vi "DriveConfigConvert.vi"(4 "Static Drive Configuration in":T1={"Correction Gain % (CG)"=1, "Dead Band (DB)"=10, "Dead Band Window (DW)"=10, "Encoder Resolution (ER)"=4000, "Step Mode  (FSB)"=1, "Position Maintenance (FSC)"=0, "Stop on Stall (FSD)"=1, "Activate OP1 on stall (FSE)"=0, "Stop on Trigger 3 (FSF)"=0, "OP2 in Deadband (FSG)"=0, "Stall Detect (FSH)"=1, "Limit Disable (LD)"=0, "Motor Resolution (MR)"=enum."20000", "Limit Switch Sense (OSA)"=0, "Home Position (OSB)"=1, "Home Switch Sense (OSC)"=0, "Encoder Z for Home (OSD)"=1, "Reference edge of Home (OSH)"=0, "RS232 Echo Control (SSA)"=0, "Buffer at Limit (SSG)"=1, "Buffer at Stop (SSH)"=1, "Indexer Mode  (FSA)"=1, "Type"="", "ConfigString"="", "De Power Motor"=enum."FALSE"} {"Indexer Mode  (FSA)" items=["Incremental", "Absolute"]; "Buffer at Stop (SSH)" items=["Clear buffer", "Save and Continue"]; "Buffer at Limit (SSG)" items=["Clear buffer", "Save and Continue"]; "RS232 Echo Control (SSA)" items=["Echo ON", "Echo OFF"]; "Reference edge of Home (OSH)" items=["CW", "CCW"]; "Encoder Z for Home (OSD)" items=["Don't use", "Enable"]; "Home Switch Sense (OSC)" items=["Normally Open", "Normally Closed"]; "Home Position (OSB)" items=["Anywhere in Switch", "Edge of Switch"]; "Limit Switch Sense (OSA)" items=["Normally Closed", "Normally Open"]; "Limit Disable (LD)" items=["Both Enabled", "CW Disabled", "CCW Disabled", "Both Disabled"]; "Stall Detect (FSH)" items=["Disable", "Enable"]; "OP2 in Deadband (FSG)" items=["Don't Use", "ACTIVATE"]; "Stop on Trigger 3 (FSF)" items=["Ignore", "STOP!"]; "Activate OP1 on stall (FSE)" items=["Do not Activate", "ACTIVATE!"]; "Stop on Stall (FSD)" items=["Continue", "STOP"]; "Position Maintenance (FSC)" items=["Disabled", "Enabled"]; "Step Mode  (FSB)" items=["Motor", "Encoder"]; "Encoder Resolution (ER)" min=1 max=50000; "Dead Band Window (DW)" min=0 max=999999999; "Dead Band (DB)" min=0 max=999999999; "Correction Gain % (CG)" items=["n/a", "12.5", "25", "37.5", "50", "62.5", "75", "87.5", "100"]}, 5 "Values in":string[](array[string]), 6 "Ch names In":string[](array[string]), 7 "Mode":enum16{"Cluster to String", "String to Cluster"}(ring)) -> (0 "Static Drive Configuration Out":T1={"Correction Gain % (CG)"=1, "Dead Band (DB)"=10, "Dead Band Window (DW)"=10, "Encoder Resolution (ER)"=4000, "Step Mode  (FSB)"=1, "Position Maintenance (FSC)"=0, "Stop on Stall (FSD)"=1, "Activate OP1 on stall (FSE)"=0, "Stop on Trigger 3 (FSF)"=0, "OP2 in Deadband (FSG)"=0, "Stall Detect (FSH)"=1, "Limit Disable (LD)"=0, "Motor Resolution (MR)"=enum."20000", "Limit Switch Sense (OSA)"=0, "Home Position (OSB)"=1, "Home Switch Sense (OSC)"=0, "Encoder Z for Home (OSD)"=1, "Reference edge of Home (OSH)"=0, "RS232 Echo Control (SSA)"=0, "Buffer at Limit (SSG)"=1, "Buffer at Stop (SSH)"=1, "Indexer Mode  (FSA)"=1, "Type"="", "ConfigString"="", "De Power Motor"=enum."FALSE"} {"Indexer Mode  (FSA)" items=["Incremental", "Absolute"]; "Buffer at Stop (SSH)" items=["Clear buffer", "Save and Continue"]; "Buffer at Limit (SSG)" items=["Clear buffer", "Save and Continue"]; "RS232 Echo Control (SSA)" items=["Echo ON", "Echo OFF"]; "Reference edge of Home (OSH)" items=["CW", "CCW"]; "Encoder Z for Home (OSD)" items=["Don't use", "Enable"]; "Home Switch Sense (OSC)" items=["Normally Open", "Normally Closed"]; "Home Position (OSB)" items=["Anywhere in Switch", "Edge of Switch"]; "Limit Switch Sense (OSA)" items=["Normally Closed", "Normally Open"]; "Limit Disable (LD)" items=["Both Enabled", "CW Disabled", "CCW Disabled", "Both Disabled"]; "Stall Detect (FSH)" items=["Disable", "Enable"]; "OP2 in Deadband (FSG)" items=["Don't Use", "ACTIVATE"]; "Stop on Trigger 3 (FSF)" items=["Ignore", "STOP!"]; "Activate OP1 on stall (FSE)" items=["Do not Activate", "ACTIVATE!"]; "Stop on Stall (FSD)" items=["Continue", "STOP"]; "Position Maintenance (FSC)" items=["Disabled", "Enabled"]; "Step Mode  (FSB)" items=["Motor", "Encoder"]; "Encoder Resolution (ER)" min=1 max=50000; "Dead Band Window (DW)" min=0 max=999999999; "Dead Band (DB)" min=0 max=999999999; "Correction Gain % (CG)" items=["n/a", "12.5", "25", "37.5", "50", "62.5", "75", "87.5", "100"]}, 1 "String Values":string[](array[string]), 2 "Ch names":string[](array[string]), 3 "Pulses/Rev":i32)   [LabVIEW 2010]
uses:
  DriveStaticConfig.ctl
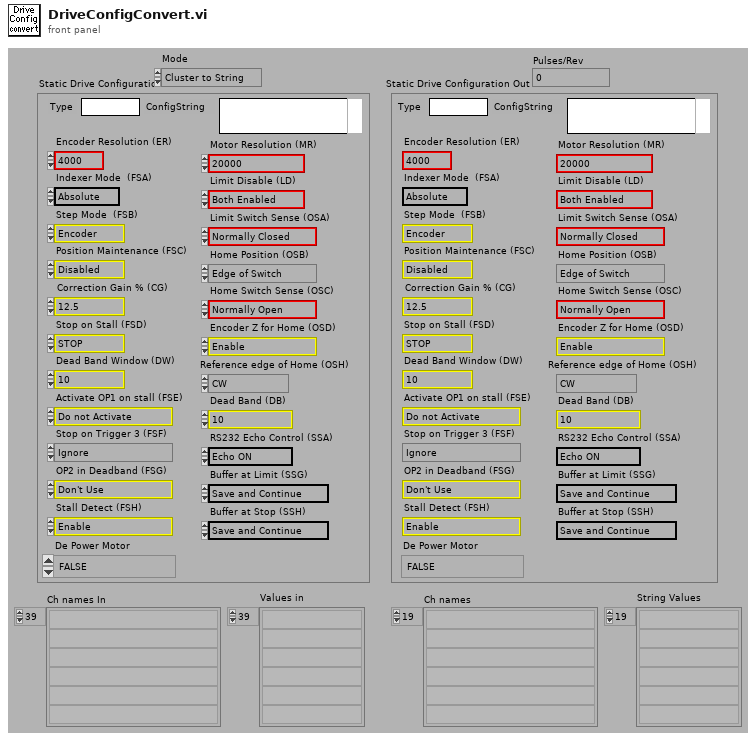
[diagram p1: front panel]
types:
  T1 = typedef "DriveStaticConfig.ctl" = cluster{"Correction Gain % (CG)":u16, "Dead Band (DB)":i32, "Dead Band Window (DW)":i32, "Encoder Resolution (ER)":i32, "Step Mode  (FSB)":u16, "Position Maintenance (FSC)":u16, "Stop on Stall (FSD)":u16, "Activate OP1 on stall (FSE)":u16, "Stop on Trigger 3 (FSF)":u16, "OP2 in Deadband (FSG)":u16, "Stall Detect (FSH)":u16, "Limit Disable (LD)":u16, "Motor Resolution (MR)":enum16{"200", "400", "1000", "2000", "4000", "5000", "10000", "12800", "18000", "20000", "21600", "25000", "25400", "25600", "36000", "50000", "278528", "425984", "507904", "614400", "655360", "819200", "1024000"}, "Limit Switch Sense (OSA)":u16, "Home Position (OSB)":u16, "Home Switch Sense (OSC)":u16, "Encoder Z for Home (OSD)":u16, "Reference edge of Home (OSH)":u16, "RS232 Echo Control (SSA)":u16, "Buffer at Limit (SSG)":u16, "Buffer at Stop (SSH)":u16, "Indexer Mode  (FSA)":u16, "Type":string, "ConfigString":string, "De Power Motor":enum16{"TRUE", "FALSE"}}
  T2 = enum16{"200", "400", "1000", "2000", "4000", "5000", "10000", "12800", "18000", "20000", "21600", "25000", "25400", "25600", "36000", "50000", "278528", "425984", "507904", "614400", "655360", "819200", "1024000"}
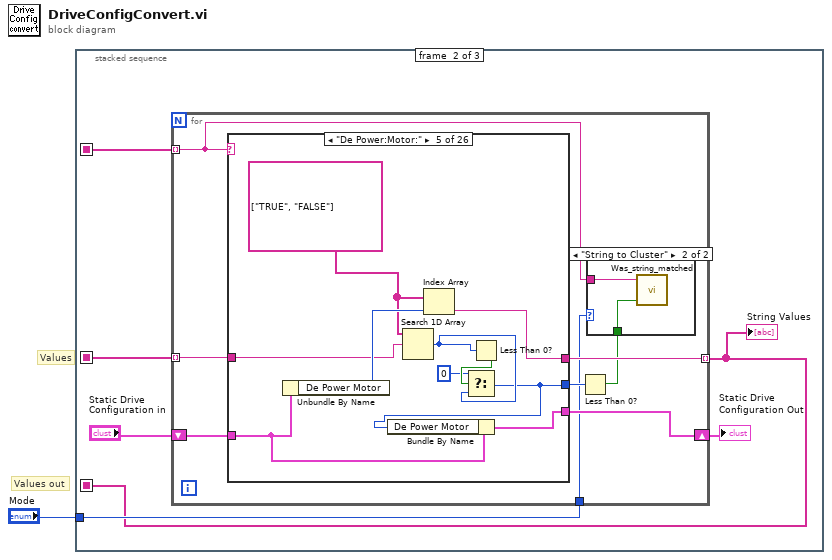
[diagram p0: block diagram]
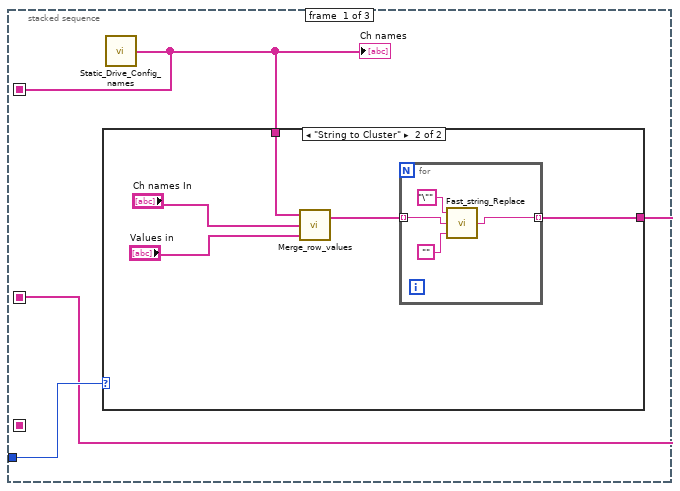
[diagram p2: hidden frame]
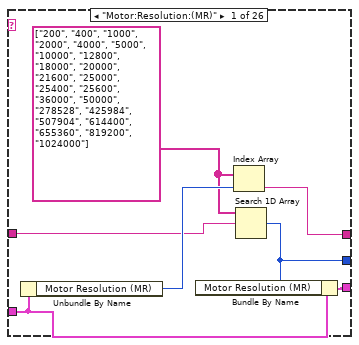
[diagram p5: hidden frame]
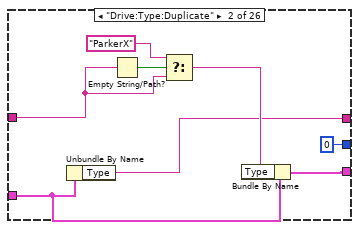
[diagram p6: hidden frame]
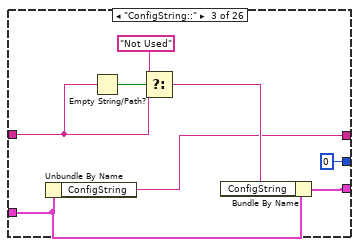
[diagram p7: hidden frame]
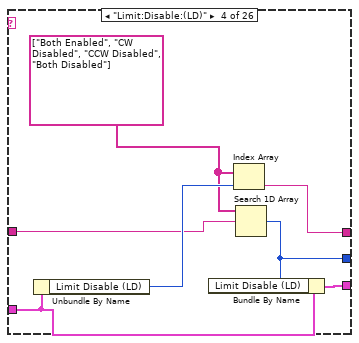
[diagram p8: hidden frame]
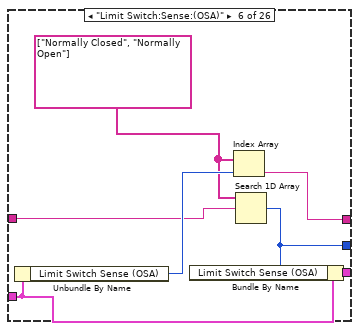
[diagram p9: hidden frame]
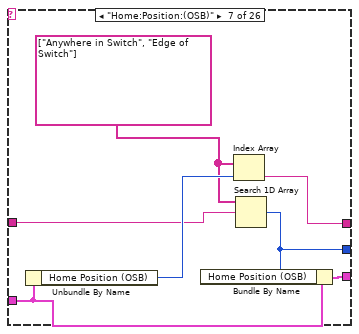
[diagram p10: hidden frame]
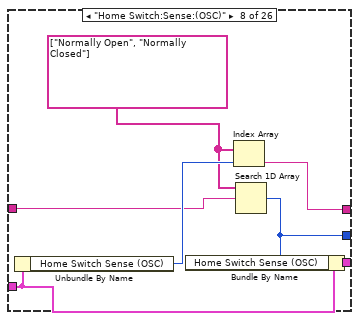
[diagram p11: hidden frame]
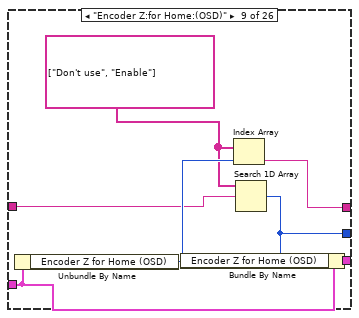
[diagram p12: hidden frame]
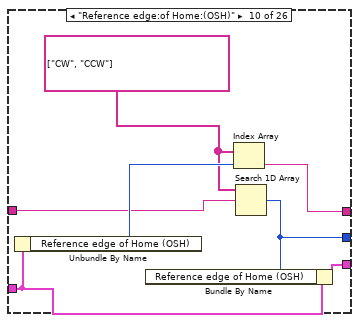
[diagram p13: hidden frame]
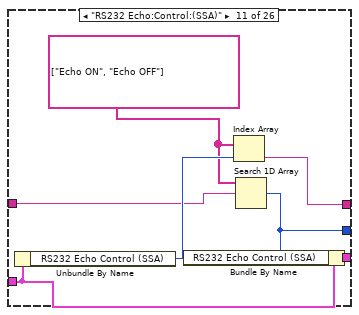
[diagram p14: hidden frame]
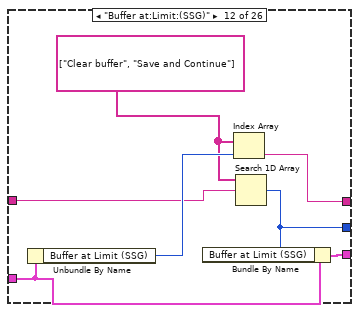
[diagram p15: hidden frame]
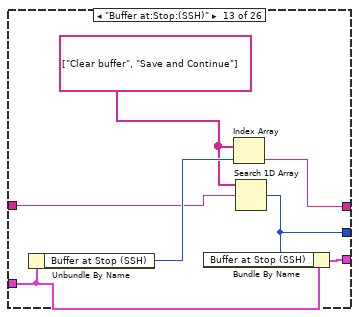
[diagram p16: hidden frame]
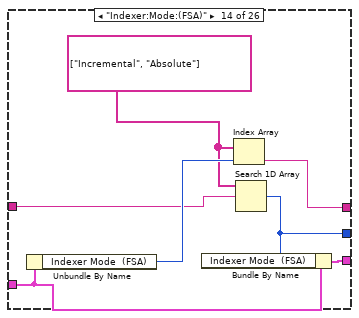
[diagram p17: hidden frame]
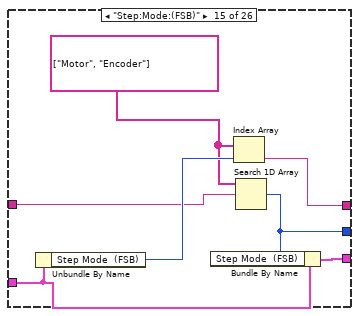
[diagram p18: hidden frame]
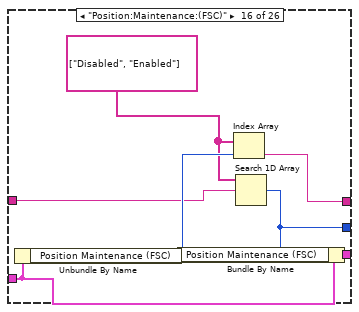
[diagram p19: hidden frame]
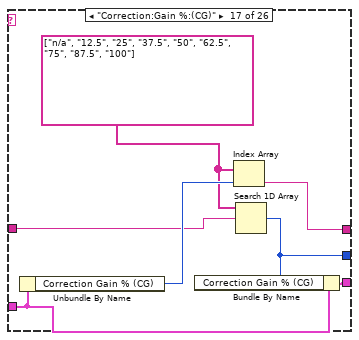
[diagram p20: hidden frame]
diagram:
  # "Values out"
  # "Values"
  n1 = stacked-sequence {
    seq-local: [w3 _ _] -> [_ w17 w222]
    seq-local: [w2 _ _] -> [_ w16 w216]
    seq-local: [_ w15 _] -> [_ _ w223]
    tunnel: "Mode" -> [w4 w18 w225]
    frame #0 {
      n2 = call "Static_Drive_Config_names.vi"() -> ("Ch names"=w2:string[])
      "Ch names" <- w2
      n3 = case shown="\"String to Cluster\"" w4 {
        tunnel: [w5 w6] -> w3
        tunnel: w2 -> [w5 w8]
        frame "Cluster to String" {
        }
        frame "String to Cluster" {
          n4 = call "Merge_row_values.vi"("Present Row values"="Values in", "Present Channels"="Ch names In", "Desired Channels"=w8) -> ("Desired Row values"=w7:string[])  [unwired: 1 out]
          n5 = for {
            tunnel: w7 -> [w14] mode=indexing
            tunnel: [w13] -> w6 mode=indexing
            n6 = call "Fast_string_Replace.vi"("Replace match with:"="", "Input String"=w14, "regular expression"="\"") -> ("Output String"=w13:string)  [unwired: 2 out]
          }
        }
      }
    }
    frame #1 {
      n7 = for {
        tunnel: w16 -> [w22] mode=indexing
        shift-right: [w25] -> w19
        shift-left: "Static Drive Configuration in" -> [w28]
        tunnel: [w27] -> w15 mode=indexing
        tunnel: w17 -> [w26] mode=indexing
        tunnel: w18 -> [w21]
        n8 = case shown="\"De Power:Motor:\"" w22 {
          tunnel: w28 -> [w37 w45 w53 w60 w70 w77 w84 w91 w98 w105 w112 w119 w126 w133 w140 w147 w154 w161 w168 w175 w182 w189 w194 w201 w208 w212]
          tunnel: [w35 w38 w47 w58 w68 w75 w82 w89 w96 w103 w110 w117 w124 w131 w138 w145 w152 w159 w166 w173 w180 w187 w195 w202 w209 ""] -> w27
          tunnel: w26 -> [w34 w41 w50 w57 w67 w74 w81 w88 w95 w102 w109 w116 w123 w130 w137 w144 w151 w158 w165 w172 w179 w186 w192 w199 w206 _]
          tunnel: [w33 w44 w52 w56 w66 w73 w80 w87 w94 w101 w108 w115 w122 w129 w136 w143 w150 w157 w164 w171 w178 w185 w193 w200 w207 w212] -> w25
          tunnel: [w32 0 ("index of element") 0 ("index of element") w55 w61 w72 w79 w86 w93 w100 w107 w114 w121 w128 w135 w142 w149 w156 w163 w170 w177 w184 0 ("index of element") 0 ("index of element") 0 ("index of element") -1 ("index of element")] -> w24
          frame "Motor:Resolution:(MR)" {
            w31 = string[] ["200", "400", "1000", "2000", "4000", "5000", "10000", "12800", "18000", "20000", "21600", "25000", "25400", "25600", "36000", "50000", "278528", "425984", "507904", "614400", "655360", "819200", "1024000"] ("Write Attribute")
            n9 = Unbundle By Name(w37) -> ("Motor Resolution (MR)"=w36:T2)
            n10 = Index Array(array=w31, index=w36) -> (element=w35:string)
            n11 = Search 1D Array(1D array=w31, element=w34) -> (index of element=w32:i32)  [unwired: 1 out]
            n12 = Bundle By Name(cluster=w37, "Motor Resolution (MR)"=w32) -> (w33:T1)
          }
          frame "Drive:Type:Duplicate" {
            n13 = Unbundle By Name(w45) -> ("Type"=w38:string)
            n14 = Empty String/Path?(string/path=w41) -> (empty?=w43:bool)
            n15 = Select(t="ParkerX", s=w43, f=w41) -> (s? t:f=w40:string)
            n16 = Bundle By Name(cluster=w45, "Type"=w40) -> (w44:T1)
          }
          frame "ConfigString::" {
            n17 = Unbundle By Name(w53) -> ("ConfigString"=w47:string)
            n18 = Empty String/Path?(string/path=w50) -> (empty?=w51:bool)
            n19 = Select(t="Not Used", s=w51, f=w50) -> (s? t:f=w49:string)
            n20 = Bundle By Name(cluster=w53, "ConfigString"=w49) -> (w52:T1)
          }
          frame "Limit:Disable:(LD)" {
            w54 = string[] ["Both Enabled", "CW Disabled", "CCW Disabled", "Both Disabled"] ("Read Attribute")
            n21 = Unbundle By Name(w60) -> ("Limit Disable (LD)"=w59:u16)
            n22 = Index Array(array=w54, index=w59) -> (element=w58:string)
            n23 = Search 1D Array(1D array=w54, element=w57) -> (index of element=w55:i32)  [unwired: 1 out]
            n24 = Bundle By Name(cluster=w60, "Limit Disable (LD)"=w55) -> (w56:T1)
          }
          frame "De Power:Motor:" {
            w65 = string[] ["TRUE", "FALSE"] ("Read Attribute")
            n25 = Unbundle By Name(w70) -> ("De Power Motor"=w69:enum16{"TRUE", "FALSE"})
            n26 = Search 1D Array(1D array=w65, element=w67) -> (index of element=w63:i32)  [unwired: 1 out]
            n27 = Index Array(array=w65, index=w69) -> (element=w68:string)
            n28 = Less Than 0?(x=w63) -> (x < 0?=w64:bool)
            n29 = Select(t=0, s=w64, f=w63) -> (s? t:f=w61:i32)
            n30 = Bundle By Name(cluster=w70, "De Power Motor"=w61) -> (w66:T1)
          }
          frame "Limit Switch:Sense:(OSA)" {
            w71 = string[] ["Normally Closed", "Normally Open"] ("Read Attribute")
            n31 = Unbundle By Name(w77) -> ("Limit Switch Sense (OSA)"=w76:u16)
            n32 = Index Array(array=w71, index=w76) -> (element=w75:string)
            n33 = Search 1D Array(1D array=w71, element=w74) -> (index of element=w72:i32)  [unwired: 1 out]
            n34 = Bundle By Name(cluster=w77, "Limit Switch Sense (OSA)"=w72) -> (w73:T1)
          }
          frame "Home:Position:(OSB)" {
            w78 = string[] ["Anywhere in Switch", "Edge of Switch"] ("Read Attribute")
            n35 = Unbundle By Name(w84) -> ("Home Position (OSB)"=w83:u16)
            n36 = Index Array(array=w78, index=w83) -> (element=w82:string)
            n37 = Search 1D Array(1D array=w78, element=w81) -> (index of element=w79:i32)  [unwired: 1 out]
            n38 = Bundle By Name(cluster=w84, "Home Position (OSB)"=w79) -> (w80:T1)
          }
          frame "Home Switch:Sense:(OSC)" {
            w85 = string[] ["Normally Open", "Normally Closed"] ("Read Attribute")
            n39 = Unbundle By Name(w91) -> ("Home Switch Sense (OSC)"=w90:u16)
            n40 = Index Array(array=w85, index=w90) -> (element=w89:string)
            n41 = Search 1D Array(1D array=w85, element=w88) -> (index of element=w86:i32)  [unwired: 1 out]
            n42 = Bundle By Name(cluster=w91, "Home Switch Sense (OSC)"=w86) -> (w87:T1)
          }
          frame "Encoder Z:for Home:(OSD)" {
            w92 = string[] ["Don't use", "Enable"] ("Read Attribute")
            n43 = Unbundle By Name(w98) -> ("Encoder Z for Home (OSD)"=w97:u16)
            n44 = Index Array(array=w92, index=w97) -> (element=w96:string)
            n45 = Search 1D Array(1D array=w92, element=w95) -> (index of element=w93:i32)  [unwired: 1 out]
            n46 = Bundle By Name(cluster=w98, "Encoder Z for Home (OSD)"=w93) -> (w94:T1)
          }
          frame "Reference edge:of Home:(OSH)" {
            w99 = string[] ["CW", "CCW"] ("Read Attribute")
            n47 = Unbundle By Name(w105) -> ("Reference edge of Home (OSH)"=w104:u16)
            n48 = Index Array(array=w99, index=w104) -> (element=w103:string)
            n49 = Search 1D Array(1D array=w99, element=w102) -> (index of element=w100:i32)  [unwired: 1 out]
            n50 = Bundle By Name(cluster=w105, "Reference edge of Home (OSH)"=w100) -> (w101:T1)
          }
          frame "RS232 Echo:Control:(SSA)" {
            w106 = string[] ["Echo ON", "Echo OFF"] ("Read Attribute")
            n51 = Unbundle By Name(w112) -> ("RS232 Echo Control (SSA)"=w111:u16)
            n52 = Index Array(array=w106, index=w111) -> (element=w110:string)
            n53 = Search 1D Array(1D array=w106, element=w109) -> (index of element=w107:i32)  [unwired: 1 out]
            n54 = Bundle By Name(cluster=w112, "RS232 Echo Control (SSA)"=w107) -> (w108:T1)
          }
          frame "Buffer at:Limit:(SSG)" {
            w113 = string[] ["Clear buffer", "Save and Continue"] ("Read Attribute")
            n55 = Unbundle By Name(w119) -> ("Buffer at Limit (SSG)"=w118:u16)
            n56 = Index Array(array=w113, index=w118) -> (element=w117:string)
            n57 = Search 1D Array(1D array=w113, element=w116) -> (index of element=w114:i32)  [unwired: 1 out]
            n58 = Bundle By Name(cluster=w119, "Buffer at Limit (SSG)"=w114) -> (w115:T1)
          }
          frame "Buffer at:Stop:(SSH)" {
            w120 = string[] ["Clear buffer", "Save and Continue"] ("Read Attribute")
            n59 = Unbundle By Name(w126) -> ("Buffer at Stop (SSH)"=w125:u16)
            n60 = Index Array(array=w120, index=w125) -> (element=w124:string)
            n61 = Search 1D Array(1D array=w120, element=w123) -> (index of element=w121:i32)  [unwired: 1 out]
            n62 = Bundle By Name(cluster=w126, "Buffer at Stop (SSH)"=w121) -> (w122:T1)
          }
          frame "Indexer:Mode:(FSA)" {
            w127 = string[] ["Incremental", "Absolute"] ("Read Attribute")
            n63 = Unbundle By Name(w133) -> ("Indexer Mode  (FSA)"=w132:u16)
            n64 = Index Array(array=w127, index=w132) -> (element=w131:string)
            n65 = Search 1D Array(1D array=w127, element=w130) -> (index of element=w128:i32)  [unwired: 1 out]
            n66 = Bundle By Name(cluster=w133, "Indexer Mode  (FSA)"=w128) -> (w129:T1)
          }
          frame "Step:Mode:(FSB)" {
            w134 = string[] ["Motor", "Encoder"] ("Read Attribute")
            n67 = Unbundle By Name(w140) -> ("Step Mode  (FSB)"=w139:u16)
            n68 = Index Array(array=w134, index=w139) -> (element=w138:string)
            n69 = Search 1D Array(1D array=w134, element=w137) -> (index of element=w135:i32)  [unwired: 1 out]
            n70 = Bundle By Name(cluster=w140, "Step Mode  (FSB)"=w135) -> (w136:T1)
          }
          frame "Position:Maintenance:(FSC)" {
            w141 = string[] ["Disabled", "Enabled"] ("Read Attribute")
            n71 = Unbundle By Name(w147) -> ("Position Maintenance (FSC)"=w146:u16)
            n72 = Index Array(array=w141, index=w146) -> (element=w145:string)
            n73 = Search 1D Array(1D array=w141, element=w144) -> (index of element=w142:i32)  [unwired: 1 out]
            n74 = Bundle By Name(cluster=w147, "Position Maintenance (FSC)"=w142) -> (w143:T1)
          }
          frame "Correction:Gain %:(CG)" {
            w148 = string[] ["n/a", "12.5", "25", "37.5", "50", "62.5", "75", "87.5", "100"] ("Read Attribute")
            n75 = Unbundle By Name(w154) -> ("Correction Gain % (CG)"=w153:u16)
            n76 = Index Array(array=w148, index=w153) -> (element=w152:string)
            n77 = Search 1D Array(1D array=w148, element=w151) -> (index of element=w149:i32)  [unwired: 1 out]
            n78 = Bundle By Name(cluster=w154, "Correction Gain % (CG)"=w149) -> (w150:T1)
          }
          frame "Activate OP1:on stall:(FSE)" {
            w155 = string[] ["Do not Activate", "ACTIVATE!"] ("Read Attribute")
            n79 = Unbundle By Name(w161) -> ("Activate OP1 on stall (FSE)"=w160:u16)
            n80 = Index Array(array=w155, index=w160) -> (element=w159:string)
            n81 = Search 1D Array(1D array=w155, element=w158) -> (index of element=w156:i32)  [unwired: 1 out]
            n82 = Bundle By Name(cluster=w161, "Activate OP1 on stall (FSE)"=w156) -> (w157:T1)
          }
          frame "Stop on:Stall:(FSD)" {
            w162 = string[] ["Continue", "STOP"] ("Read Attribute")
            n83 = Unbundle By Name(w168) -> ("Stop on Stall (FSD)"=w167:u16)
            n84 = Index Array(array=w162, index=w167) -> (element=w166:string)
            n85 = Search 1D Array(1D array=w162, element=w165) -> (index of element=w163:i32)  [unwired: 1 out]
            n86 = Bundle By Name(cluster=w168, "Stop on Stall (FSD)"=w163) -> (w164:T1)
          }
          frame "OP2 in:Deadband:(FSG)" {
            w169 = string[] ["Don't Use", "ACTIVATE"] ("Read Attribute")
            n87 = Unbundle By Name(w175) -> ("OP2 in Deadband (FSG)"=w174:u16)
            n88 = Index Array(array=w169, index=w174) -> (element=w173:string)
            n89 = Search 1D Array(1D array=w169, element=w172) -> (index of element=w170:i32)  [unwired: 1 out]
            n90 = Bundle By Name(cluster=w175, "OP2 in Deadband (FSG)"=w170) -> (w171:T1)
          }
          frame "Stall:Detect:(FSH)" {
            w176 = string[] ["Disable", "Enable"] ("Read Attribute")
            n91 = Unbundle By Name(w182) -> ("Stall Detect (FSH)"=w181:u16)
            n92 = Index Array(array=w176, index=w181) -> (element=w180:string)
            n93 = Search 1D Array(1D array=w176, element=w179) -> (index of element=w177:i32)  [unwired: 1 out]
            n94 = Bundle By Name(cluster=w182, "Stall Detect (FSH)"=w177) -> (w178:T1)
          }
          frame "Stop on:Trigger 3:(FSF)" {
            w183 = string[] ["Ignore", "STOP!"] ("Read Attribute")
            n95 = Unbundle By Name(w189) -> ("Stop on Trigger 3 (FSF)"=w188:u16)
            n96 = Index Array(array=w183, index=w188) -> (element=w187:string)
            n97 = Search 1D Array(1D array=w183, element=w186) -> (index of element=w184:i32)  [unwired: 1 out]
            n98 = Bundle By Name(cluster=w189, "Stop on Trigger 3 (FSF)"=w184) -> (w185:T1)
          }
          frame "Encoder:Resolution:(ER)" {
            n99 = Unbundle By Name(w194) -> ("Encoder Resolution (ER)"=w196:i32)
            n100 = Decimal String To Number(string=w192) -> (number=w191:i32)  [unwired: 3 out]
            n101 = Number To Decimal String(number=w196) -> (decimal integer string=w195:string)  [unwired: 1 out]
            n102 = Bundle By Name(cluster=w194, "Encoder Resolution (ER)"=w191) -> (w193:T1)
          }
          frame "Dead Band:Window:(DW)" {
            n103 = Unbundle By Name(w201) -> ("Dead Band Window (DW)"=w203:i32)
            n104 = Decimal String To Number(string=w199) -> (number=w198:i32)  [unwired: 3 out]
            n105 = Number To Decimal String(number=w203) -> (decimal integer string=w202:string)  [unwired: 1 out]
            n106 = Bundle By Name(cluster=w201, "Dead Band Window (DW)"=w198) -> (w200:T1)
          }
          frame "Dead:Band:(DB)" {
            n107 = Unbundle By Name(w208) -> ("Dead Band (DB)"=w210:i32)
            n108 = Decimal String To Number(string=w206) -> (number=w205:i32)  [unwired: 3 out]
            n109 = Number To Decimal String(number=w210) -> (decimal integer string=w209:string)  [unwired: 1 out]
            n110 = Bundle By Name(cluster=w208, "Dead Band (DB)"=w205) -> (w207:T1)
          }
          frame "No match", Default {
          }
        }
        n111 = Less Than 0?(x=w24) -> (x < 0?=w23:bool)
        n112 = case shown="\"String to Cluster\"" w21 {
          tunnel: w23 -> [_ w30]
          tunnel: w22 -> [_ w29]
          frame "Cluster to String" {
          }
          frame "String to Cluster" {
            n113 = call "Was_string_matched.vi"("Match Error"=w30, "Variable name"=w29) -> ()  [unwired: 1 in]
          }
        }
      }
      "Static Drive Configuration Out" <- w19
      "String Values" <- w15
    }
    frame #2 {
      n114 = case shown="\"Cluster to String\"" w225 {
        tunnel: [w232 w233] -> w219
        tunnel: w223 -> [w232 _]
        tunnel: w222 -> [_ w233]
        frame "Cluster to String" {
        }
        frame "String to Cluster" {
        }
      }
      n115 = Search 1D Array(1D array=w216, element="Step:Mode:(FSB)") -> (index of element=w224:i32)  [unwired: 1 out]
      n116 = Index Array(array=w219, index=w224) -> (element=w220:string)
      n117 = Concatenate Strings(w220, ":Resolution:") -> (w214:string)
      n118 = while {
        tunnel: w214 -> [w228]
        tunnel: [w229] -> w215
        tunnel: w216 -> [w227] mode=indexing
        i -> [w229]
        stop <- w230 continue-if-true
        n119 = Match Pattern(string=w227, regular expression=w228) -> (match substring=w231:string)  [unwired: 4 out]
        n120 = Empty String/Path?(string/path=w231) -> (empty?=w230:bool)
      }
      n121 = Index Array(array=w219, index=w215) -> (element=w218:string)
      n122 = Decimal String To Number(string=w218) -> (number=→"Pulses/Rev":i32)  [unwired: 3 out]
    }
  }
